vi "FWHM.vi"(5 "End":dbl, 7 "Start":dbl, 10 "Yaxis":dbl[](array[numeric]), 11 "Xaxis":dbl[](array[numeric])) -> (3 "FWHM":dbl)   [LabVIEW 2020]
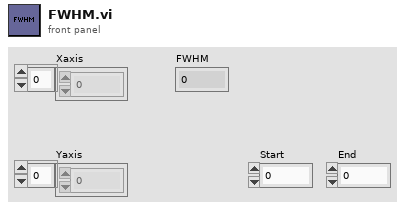
[diagram p1: front panel]
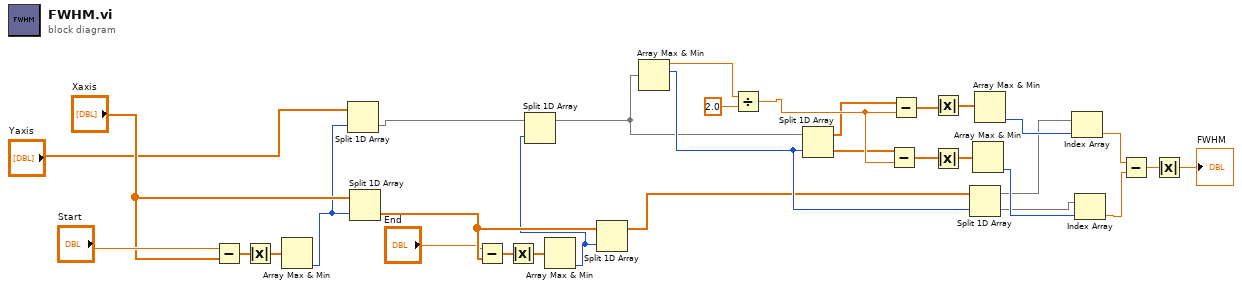
[diagram p0: block diagram]
diagram:
  n1 = Subtract(x="Start", y="Xaxis") -> (x-y=w14:dbl[])
  n2 = Absolute Value(x=w14) -> (abs(x)=w13:dbl[])
  n3 = Array Max & Min(array=w13) -> (min index (indices)=w4:i32)  [unwired: 3 out]
  n4 = Split 1D Array(array="Yaxis", index=w4) -> (second subarray=w3:dbl[])  [unwired: 1 out]
  n5 = Split 1D Array(array="Xaxis", index=w4) -> (second subarray=w10:dbl[])  [unwired: 1 out]
  n6 = Subtract(x="End", y=w10) -> (x-y=w12:dbl[])
  n7 = Absolute Value(x=w12) -> (abs(x)=w11:dbl[])
  n8 = Array Max & Min(array=w11) -> (min index (indices)=w2:i32)  [unwired: 3 out]
  n9 = Split 1D Array(array=w3, index=w2) -> (first subarray=w1:dbl[])  [unwired: 1 out]
  n10 = Split 1D Array(array=w10, index=w2) -> (first subarray=w6:dbl[])  [unwired: 1 out]
  n11 = Array Max & Min(array=w1) -> (max value=w15:dbl, max index (indices)=w32:i32)  [unwired: 2 out]
  n12 = Divide(x=w15, y=2.0) -> (x/y=w19:dbl)
  n13 = Split 1D Array(array=w1, index=w32) -> (first subarray=w17:dbl[], second subarray=w18:dbl[])
  n14 = Subtract(x=w18, y=w19) -> (x-y=w21:dbl[])
  n15 = Subtract(x=w17, y=w19) -> (x-y=w20:dbl[])
  n16 = Absolute Value(x=w20) -> (abs(x)=w22:dbl[])
  n17 = Absolute Value(x=w21) -> (abs(x)=w23:dbl[])
  n18 = Split 1D Array(array=w6, index=w32) -> (first subarray=w24:dbl[], second subarray=w26:dbl[])
  n19 = Array Max & Min(array=w23) -> (min index (indices)=w27:i32)  [unwired: 3 out]
  n20 = Array Max & Min(array=w22) -> (min index (indices)=w25:i32)  [unwired: 3 out]
  n21 = Index Array(array=w24, index=w25) -> (element=w29:dbl)
  n22 = Index Array(array=w26, index=w27) -> (element=w30:dbl)
  n23 = Subtract(x=w29, y=w30) -> (x-y=w28:dbl)
  n24 = Absolute Value(x=w28) -> (abs(x)=→"FWHM":dbl)
